vi "G_ref.vi"(3 "error in (no error)":errorcluster, 4 "wd[k]":dbl, 5 "xd[k-1]":dbl, 6 "x[k-1]":dbl) -> (0 "error out":errorcluster, 1 "xd[k]":dbl, 2 "x[k]":dbl)   [LabVIEW 2021]
uses:
  <vilib>/ptbypt/NI_PtbyPt.lvlib
panel:
  out "bs":dbl
  out "b1":dbl
  out "b0":dbl
  out "a2":dbl
  out "a1":dbl
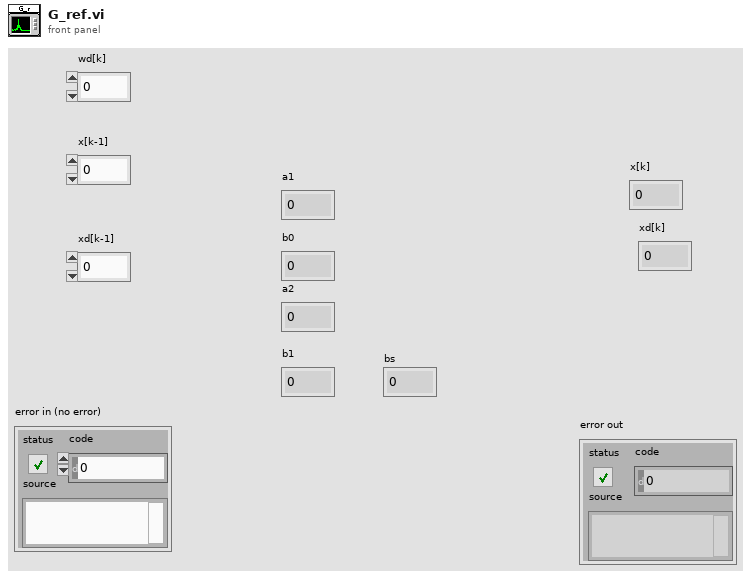
[diagram p1: front panel]
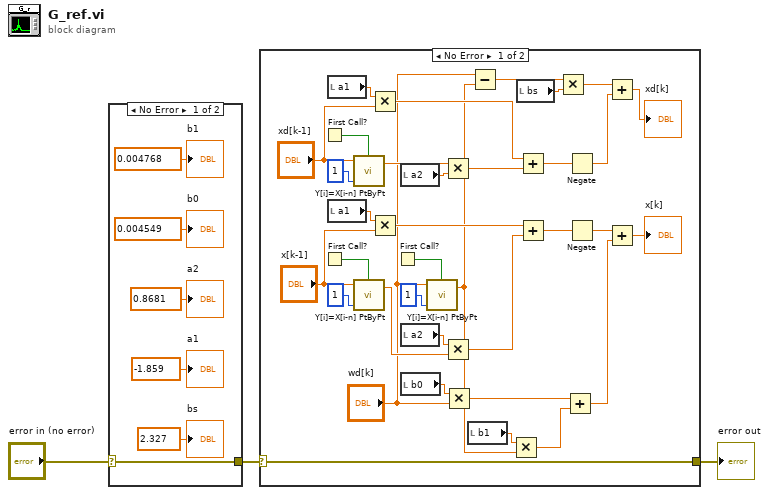
[diagram p0: block diagram]
diagram:
  n1 = case shown="No Error" "error in (no error)" {
    selector: "error in (no error)" -> [w4 w10]
    tunnel: [w4 w10] -> w2
    frame No Error {
      "a1" <- -1.859 ("Gd.a1")
      "a2" <- 0.8681 ("Gd.a2")
      "b0" <- 0.004549 ("Gd.b0")
      "b1" <- 0.004768 ("Gd.b1")
      "bs" <- 2.327 ("bs")
    }
    frame Error {
    }
  }
  n2 = case shown="No Error" w2 {
    selector: w2 -> [w11 w46]
    tunnel: [w11 w46] -> w1
    frame No Error {
      n3 = First Call?() -> (First Call?: T/F=w26:bool)
      n4 = First Call?() -> (First Call?: T/F=w40:bool)
      n5 = local read "a1"() -> (w25:dbl)
      n6 = local read "a1"() -> (w44:dbl)
      n7 = call <vilib>:"Y[i]=X[i-n] PtByPt.vi"("initialize"=w26, "shifts: n"=1, "x"="xd[k-1]") -> ("shifted x"=w22:dbl)  [unwired: 1 in, 1 out]
      n8 = call <vilib>:"Y[i]=X[i-n] PtByPt.vi"("initialize"=w40, "shifts: n"=1, "x"="x[k-1]") -> ("shifted x"=w42:dbl)  [unwired: 1 in, 1 out]
      n9 = Multiply(x=w25, y="xd[k-1]") -> (x*y=w20:dbl)
      n10 = Multiply(x=w44, y="x[k-1]") -> (x*y=w39:dbl)
      n11 = First Call?() -> (First Call?: T/F=w37:bool)
      n12 = local read "a2"() -> (w23:dbl)
      n13 = local read "a2"() -> (w41:dbl)
      n14 = local read "b0"() -> (w33:dbl)
      n15 = call <vilib>:"Y[i]=X[i-n] PtByPt.vi"("initialize"=w37, "shifts: n"=1, "x"="wd[k]") -> ("shifted x"=w17:dbl)  [unwired: 1 in, 1 out]
      n16 = Multiply(x=w22, y=w23) -> (x*y=w21:dbl)
      n17 = Multiply(x=w41, y=w42) -> (x*y=w38:dbl)
      n18 = Multiply(x=w33, y="wd[k]") -> (x*y=w31:dbl)
      n19 = local read "b1"() -> (w34:dbl)
      n20 = Subtract(x="wd[k]", y=w17) -> (x-y=w16:dbl)
      n21 = Multiply(x=w34, y=w17) -> (x*y=w32:dbl)
      n22 = local read "bs"() -> (w15:dbl)
      n23 = Add(x=w20, y=w21) -> (x+y=w19:dbl)
      n24 = Add(x=w39, y=w38) -> (x+y=w35:dbl)
      n25 = Multiply(x=w16, y=w15) -> (x*y=w13:dbl)
      n26 = Add(x=w31, y=w32) -> (x+y=w29:dbl)
      n27 = Negate(x=w19) -> (-x=w14:dbl)
      n28 = Negate(x=w35) -> (-x=w30:dbl)
      n29 = Add(x=w13, y=w14) -> (x+y=→"xd[k]":dbl)
      n30 = Add(x=w30, y=w29) -> (x+y=→"x[k]":dbl)
    }
    frame Error {
    }
  }
  "error out" <- w1
